vi "Dictionary Test - 008.vi"(8 "error in (no error)":errorcluster) -> (0 "error out":errorcluster, 2 "pass":bool)   [LabVIEW 2009]
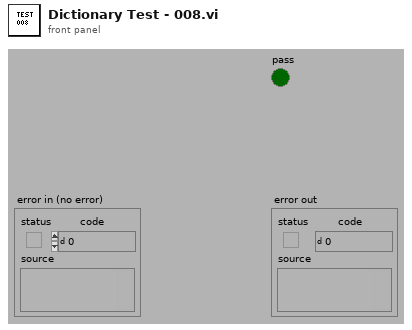
[diagram p1: front panel]
types:
  T1 = typedef "Dictionary Object RefNum.ctl" = refnum<k1>
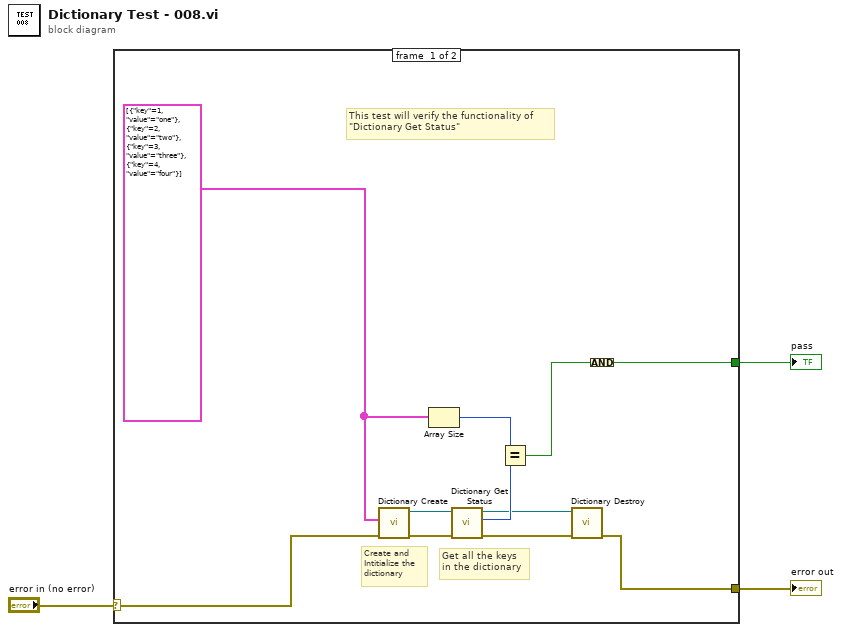
[diagram p0: block diagram]
diagram:
  n1 = case shown="No Error" "error in (no error)" {
    selector: "error in (no error)" -> [w14 w15]
    tunnel: [w13 w15] -> w1
    tunnel: [w12 _] -> w3
    frame #0 {
      w8 = cluster{"key":i32, "value":string}[] [{"key"=1, "value"="one"}, {"key"=2, "value"="two"}, {"key"=3, "value"="three"}, {"key"=4, "value"="four"}] ("dictionary with updates")
      # "Create and Intitialize the dictionary"
      # "Get all the keys \nin the dictionary"
      # "This test will verify the functionality of \n\"Dictionary Get Status\""
      n2 = call "Dictionary Create.vi"("error in (no error)"=w14, "initial dictionary (empty)"=w8) -> ("error out"=w10:errorcluster, "dictionary out"=w9:T1)  [unwired: 8 in]
      n3 = Array Size(array=w8) -> (size(s)=w7:i32)
      n4 = call "Dictionary Get Status.vi"("error in (no error)"=w10, "dictionary"=w9) -> ("error out"=w11:errorcluster, "size"=w6:i32, "dictionary out"=w5:T1)  [unwired: 7 in]
      n5 = Equal?(x=w7, y=w6) -> (x = y?=w4:bool)
      n6 = call "Dictionary Destroy.vi"("error in (no error)"=w11, "dictionary"=w5) -> ("error out"=w13:errorcluster)  [unwired: 9 in]
      n7 = Compound Arithmetic op=AND(w4) -> (w12:bool)
    }
    frame #1 {
    }
  }
  "pass" <- w3
  "error out" <- w1
